vi "GetStepIndex.vi"(8 "error in (no error)":errorcluster) -> (0 "error out":errorcluster, 2 "found":bool, 3 "Index":T1)   [LabVIEW 2016, in "SeqProcessor.lvlib"]
uses:
  SeqProcessor.lvlib
  controls/StepIndex.ctl
  <vilib>/addons/PointValueMap/subVIs/Point_Read_variant.vi
  <vilib>/addons/PointValueMap/PointValueMap.lvlib
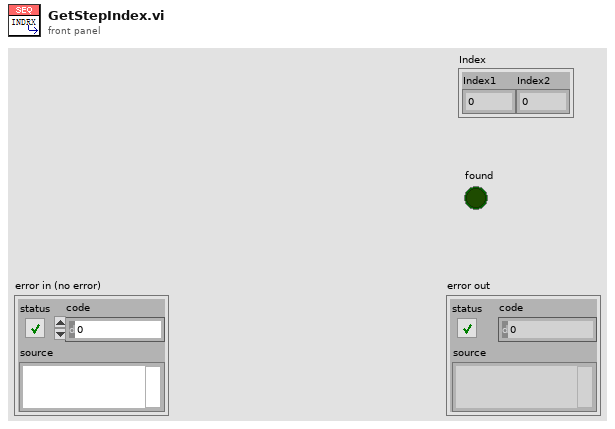
[diagram p1: front panel]
types:
  T1 = typedef "SeqProcessor.lvlib/StepIndex.ctl" = cluster{"Index1":u32, "Index2":u32}
  T2 = typedef "PointValueMap.lvlib/PointMap.ctl" = refnum<data-value>
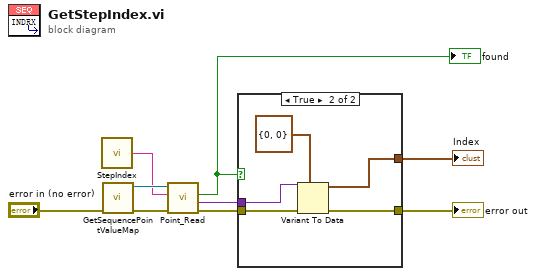
[diagram p0: block diagram]
diagram:
  n1 = call "StepIndex.vi"() -> ("StepIndex"=w3:string)  [unwired: 5 in]
  n2 = call "GetSequencePointValueMap.vi"("error in (no error)"="error in (no error)") -> ("error out"=w5:errorcluster, "SeqMap"=w4:T2)  [unwired: 9 in]
  n3 = call-poly <vilib>:"Point_Read.vi"("Error In"=w5, "Tag"=w3, "Map"=w4) -> ("Error Out"=w8:errorcluster, "Value"=w7:variant, "Found?"=w6:bool)  [unwired: 3 in, 3 out]
  "found" <- w6
  n4 = case shown="True" w6 {
    tunnel: w8 -> [w10 w15]
    tunnel: [w10 w14] -> w2
    tunnel: w7 -> [_ w13]
    tunnel: [_ w12] -> w1
    frame False {
    }
    frame True {
      n5 = Variant To Data(error in=w15, type=T1 {"Index1"=0, "Index2"=0} ("Index"), Variant=w13) -> (data=w12:T1, error out=w14:errorcluster)
    }
  }
  "error out" <- w2
  "Index" <- w1
